vi "Test Quirc QR Code Detector.vi"(11 "Test Case In":refnum<class "02_FeatureDetection.lvclass">) -> (0 "error out":errorcluster, 3 "Test Case Out":refnum<class "02_FeatureDetection.lvclass">)   [LabVIEW 2020, in "test.lvlib" / "02_FeatureDetection.lvclass"]
uses:
  02_FeatureDetection.lvclass
  C:/Program Files (x86)/National Instruments/LabVIEW 2026/vi.lib/Astemes/LUnit/Test Case.lvclass
  <vilib>/picture/picture.llb/imagedata.ctl
  feature_detection/QR Code Detector/QR Code Detector.lvclass/QR Code Detector.ctl
  <vilib>/Astemes/LUnit/Test Case.lvclass/Test Case.ctl
  image/New Image (ARGB Preallocated).vi
  image/Copy Pixmap to Image (ARGB Flatten Mask).vi
  feature_detection/QR Code Detector/Detect and Decode Multiple (ARGB).vi
  c620ff27-3bdc-43ee-ae28-79191c7efa9c.vi
  image/New Image (Greyscale Preallocated).vi
  image/Copy Pixmap to Image (Greyscale Flatten Mask).vi
  feature_detection/QR Code Detector/Detect and Decode Multiple (Greyscale).vi
  81cff08c-ad27-40c1-b34f-f5a0f1f6849e.vi
  image/New Image (ARGB Preallocated).vi/3321fa97-f432-4e1e-8db9-a0df79aed21b.vi
  image/ARGB Colour to U32 Pixel Value.vi
  image/Copy Pixmap to Image (ARGB Flatten Mask).vi/7d03ccf7-b889-4e8d-9f2a-57831e73dbde.vi
  feature_detection/QR Code Detector/Detect and Decode Multiple (ARGB).vi/844373d0-3d5f-493c-b88a-dd91dd1f862c.vi
  <vilib>/Astemes/LUnit/Core/LUnit Test Case/Private/Append Pass Result.vi
  <vilib>/Astemes/LUnit/Core/LUnit Test Case/Private/Append Fail Result.vi
  c620ff27-3bdc-43ee-ae28-79191c7efa9c.vi/9c5d11cd-9439-4240-a1ee-d9baace9c924.vi
  image/New Image (Greyscale Preallocated).vi/6598b9e0-8a08-46f5-91fd-ca1b87217137.vi
  image/Copy Pixmap to Image (Greyscale Flatten Mask).vi/f0818824-bd55-4656-87f2-fcc208e7cf24.vi
  feature_detection/QR Code Detector/Detect and Decode Multiple (Greyscale).vi/97a01b78-84de-4c9d-a407-2dc45d320d5a.vi
  81cff08c-ad27-40c1-b34f-f5a0f1f6849e.vi/9c5d11cd-9439-4240-a1ee-d9baace9c924.vi
  image/FixPixmap.vi
  <vilib>/Astemes/LUnit/Core/LUnit Test Case/Private/Run In UI.vi
  image/Default8bitColourMap.vi
  <vilib>/Utility/error.llb/Clear Errors.vi
  <vilib>/Utility/error.llb/Error Cluster From Error Code.vi
  image/image.lvlib
  feature_detection/QR Code Detector/QR Code Detector.lvclass
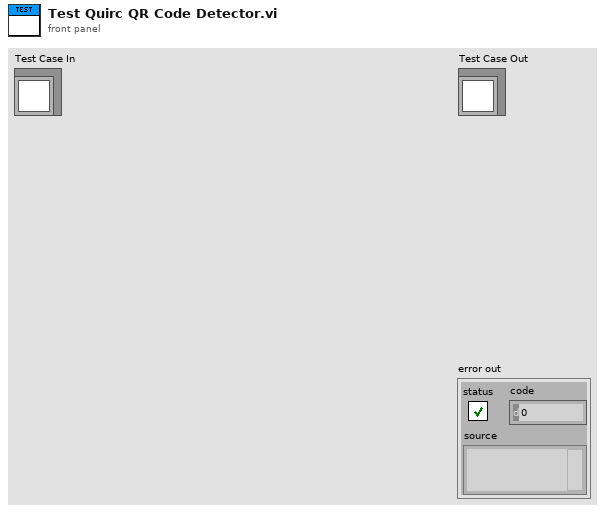
[diagram p1: front panel]
types:
  T1 = typedef "imagedata.ctl" = cluster{"image type":i32, "image depth":i32, "image":u8[], "mask":u8[], "colors":u32[], "Rectangle":cluster{"left":i16, "top":i16, "right":i16, "bottom":i16}}
  T2 = cluster{"Data":string, cluster{cluster{"x":i32, "y":i32}, cluster{"x":i32, "y":i32}, cluster{"x":i32, "y":i32}, cluster{"x":i32, "y":i32}}}[]
  T3 = typedef "image.lvlib/ARGB Image.ctl" = refnum<data-value>
  T4 = typedef "feature_detection.lvlib/QR Code Detector.lvclass/Detection.ctl" = cluster{"Data":string, "Corners":T5}
  T5 = typedef "common.lvlib/Image Points Quad (Float).ctl" = cluster{"A":T6, "B":T6, "C":T6, "D":T6}
  T6 = typedef "common.lvlib/Image Point (Float).ctl" = cluster{"x":dbl, "y":dbl}
  T7 = cluster{cluster{"x":i32, "y":i32}, cluster{"x":i32, "y":i32}, cluster{"x":i32, "y":i32}, cluster{"x":i32, "y":i32}}
  T8 = cluster{"Data":string, cluster{cluster{"x":i32, "y":i32}, cluster{"x":i32, "y":i32}, cluster{"x":i32, "y":i32}, cluster{"x":i32, "y":i32}}}
  T9 = typedef "image.lvlib/Greyscale Image.ctl" = refnum<data-value>
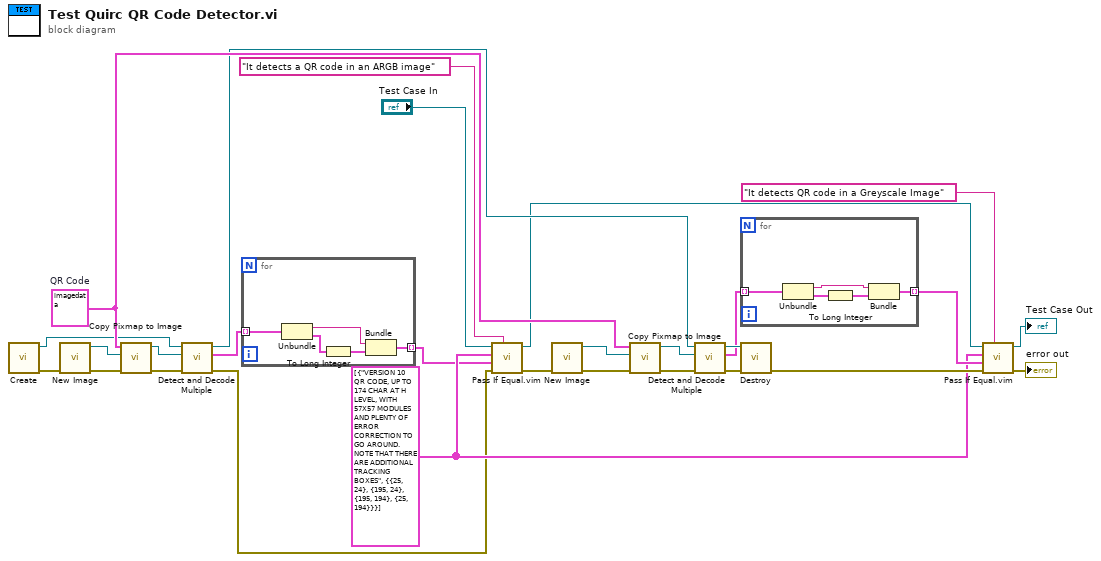
[diagram p0: block diagram]
diagram:
  w22 = T1 {"image type"=0, "image depth"=24, "image"=array[145200 elements], "mask"=[], "colors"=[], "Rectangle"={"left"=0, "top"=0, "right"=220, "bottom"=220}}  # QR Code
  w5 = T2 [{"Data"="VERSION 10 QR CODE, UP TO 174 CHAR AT H LEVEL, WITH 57X57 MODULES AND PLENTY OF ERROR CORRECTION TO GO AROUND.  NOTE THAT THERE ARE ADDITIONAL TRACKING BOXES", {{"x"=25, "y"=24}, {"x"=195, "y"=24}, {"x"=195, "y"=194}, {"x"=25, "y"=194}}}] ("Array")
  n1 = call "Create.vi"() -> ("error out"=w27:errorcluster, "QR Code Detector"=w3:refnum<class "QR Code Detector.lvclass">)  [unwired: 10 in]
  n2 = call-poly "New Image.vi"("error in (no error)"=w27) -> ("error out"=w25:errorcluster, "ARGB Image"=w26:T3)  [unwired: 9 in]
  n3 = call-poly "Copy Pixmap to Image.vi"("error in (no error)"=w25, "ARGB Image Destination in"=w26, "Pixmap Image Data"=w22) -> ("error out"=w24:errorcluster, "ARGB Image Destination"=w2:T3)  [unwired: 7 in]
  n4 = call-poly "Detect and Decode Multiple.vi"("error in (no error)"=w24, "ARGB Image in"=w2, "QR Code Detector in"=w3) -> ("error out"=w1:errorcluster, "Detections"=w8:T4[], "QR Code Detector"=w19:refnum<class "QR Code Detector.lvclass">)  [unwired: 6 in]
  n5 = for {
    tunnel: w8 -> [w33] mode=indexing
    tunnel: [w29] -> w4 mode=indexing
    n6 = Unbundle(w33) -> ("Data"=w32:string, "Corners"=w31:T5)
    n7 = To Long Integer(number=w31) -> (32bit integer=w30:T7)
    n8 = Bundle("Data"=w32, w30) -> (w29:T8)  [unwired: 1 in]
  }
  n9 = call "Pass If Equal.vim"("Description"="It detects a QR code in an ARGB image", "error in (no error)"=w1, "Actual"=w4, "Expected"=w5, "LUnit Test Case In"="Test Case In") -> ("error out"=w14:errorcluster, "LUnit Test Case Out"=w13:refnum<class "02_FeatureDetection.lvclass">)  [unwired: 5 in]
  n10 = call-poly "New Image.vi"("error in (no error)"=w14) -> ("error out"=w21:errorcluster, "Greyscale Image"=w20:T9)  [unwired: 9 in]
  n11 = call-poly "Copy Pixmap to Image.vi"("error in (no error)"=w21, "Greyscale Image Destination in"=w20, "Pixmap Image Data"=w22) -> ("error out"=w17:errorcluster, "Greyscale Image Destination"=w18:T9)  [unwired: 7 in]
  n12 = call-poly "Detect and Decode Multiple.vi"("error in (no error)"=w17, "Greyscale Image in"=w18, "QR Code Detector in"=w19) -> ("error out"=w16:errorcluster, "Detections"=w7:T4[], "QR Code Detector"=w15:refnum<class "QR Code Detector.lvclass">)  [unwired: 6 in]
  n13 = for {
    tunnel: w7 -> [w38] mode=indexing
    tunnel: [w35] -> w6 mode=indexing
    n14 = Unbundle(w38) -> ("Data"=w37:string, "Corners"=w36:T5)
    n15 = To Long Integer(number=w36) -> (32bit integer=w34:T7)
    n16 = Bundle("Data"=w37, w34) -> (w35:T8)  [unwired: 1 in]
  }
  n17 = call "Destroy.vi"("error in (no error)"=w16, "QR Code Detector in"=w15) -> ("error out"=w11:errorcluster)  [unwired: 9 in]
  n18 = call "Pass If Equal.vim"("Description"="It detects QR code in a Greyscale Image", "error in (no error)"=w11, "Actual"=w6, "Expected"=w5, "LUnit Test Case In"=w13) -> ("error out"=→"error out":errorcluster, "LUnit Test Case Out"=→"Test Case Out":refnum<class "02_FeatureDetection.lvclass">)  [unwired: 5 in]
